vi "VISet.vi"(0 "Signal":bool, 1 "data string":string, 2 "variant":variant, 3 "Name":string, 4 "VI Name":string, 5 "Options":i32=16 format="%.0x", 6 "Path":path, 7 "Port":u16=3364, 8 "Address":string="localhost") -> ()   [LabVIEW 2014]
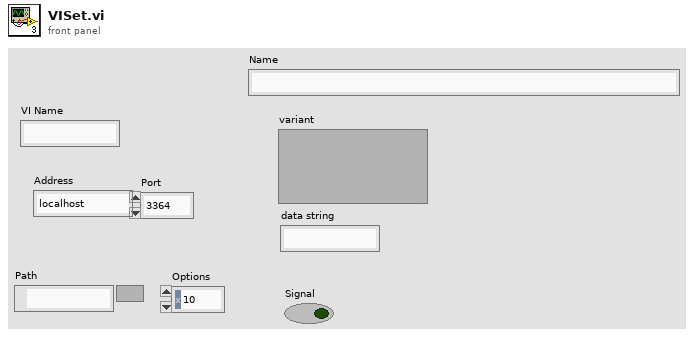
[diagram p1: front panel]
types:
  T1 = cluster{"Name":string, "Reference":refnum<vi>, "Ctrls":cluster{"Name":string, "Ctrl":refnum<vi>}[]}
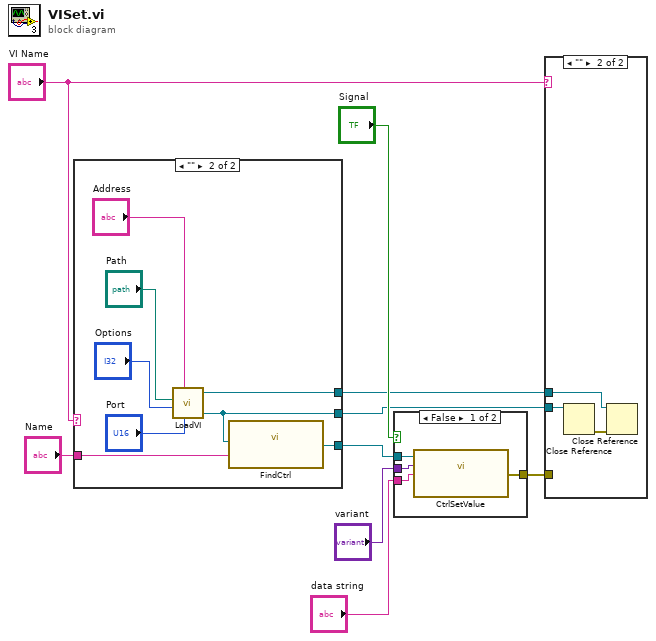
[diagram p0: block diagram]
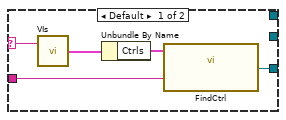
[diagram p3: hidden frame]
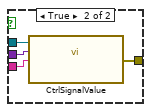
[diagram p4: hidden frame]
diagram:
  n1 = case shown="\"\"" "VI Name" {
    selector: "VI Name" -> [w14 _]
    tunnel: "Name" -> [w11 w21]
    tunnel: [w10 w22] -> w2
    tunnel: [_ w20] -> w4
    tunnel: [_ w17] -> w3
    frame Default {
      n2 = call "VIs.vi"("Name"=w14) -> ("VI Out"=w13:T1)  [unwired: 1 in]
      n3 = Unbundle By Name(w13) -> ("Ctrls"=w12:cluster{"Name":string, "Ctrl":refnum<vi>}[])
      n4 = call "FindCtrl.vi"("Name"=w11, "Ctrls"=w12) -> ("Ctrl"=w10:refnum<vi>)  [unwired: 1 in]
    }
    frame "" {
      n5 = call "LoadVI.vi"("Address"="Address", "Path"="Path", "Options"="Options", "Port"="Port") -> ("LabVIEW Out"=w17:refnum<vi>, "Reference"=w20:refnum<vi>)  [unwired: 3 in]
      n6 = call "FindCtrl.vi"("Name"=w21, "VI"=w20) -> ("Ctrl"=w22:refnum<vi>)  [unwired: 1 in]
    }
  }
  n7 = case shown="False" "Signal" {
    tunnel: w2 -> [w26 w30]
    tunnel: "variant" -> [w25 w29]
    tunnel: "data string" -> [w24 w28]
    tunnel: [w23 w27] -> w1
    frame False {
      n8 = call "CtrlSetValue.vi"("data string"=w24, "variant"=w25, "reference"=w26) -> ("error out"=w23:errorcluster)  [unwired: 1 in]
    }
    frame True {
      n9 = call "CtrlSignalValue.vi"("data string"=w28, "variant"=w29, "reference"=w30) -> ("error out"=w27:errorcluster)  [unwired: 1 in]
    }
  }
  n10 = case shown="\"\"" "VI Name" {
    tunnel: w4 -> [_ w33]
    tunnel: w3 -> [_ w31]
    tunnel: w1 -> [_ _]
    frame Default {
    }
    frame "" {
      n11 = Close Reference(reference=w33) -> (error out=w32:errorcluster)  [unwired: 1 in]
      n12 = Close Reference(reference=w31, error in (no error)=w32) -> ()  [unwired: 1 out]
    }
  }
